vi "41 Config File Write GPS Time (x64-2018).vi"(0 "GPS Time":string, 5 "GPS Date":string, 7 "Labview Time":dbl=0.1, 9 "CPU Time":dbl=0.1, 11 "Tick Count":dbl=0.1, 12 "GPS Lock":bool) -> ()   [LabVIEW 2017]
uses:
  <vilib>/Utility/config.llb/Write Key (Double).vi
  <vilib>/Utility/config.llb/Write Key (String).vi
  <vilib>/Utility/config.llb/Write Key (Boolean).vi
  <vilib>/Utility/config.llb/NI_LVConfig.lvlib
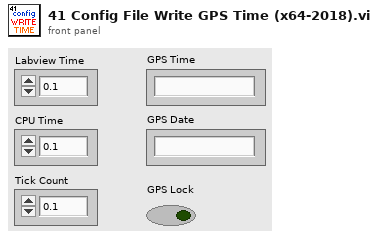
[diagram p1: front panel]
types:
  T1 = typedef "NI_LVConfig.lvlib/Config Data RefNum.ctl" = refnum<k1>
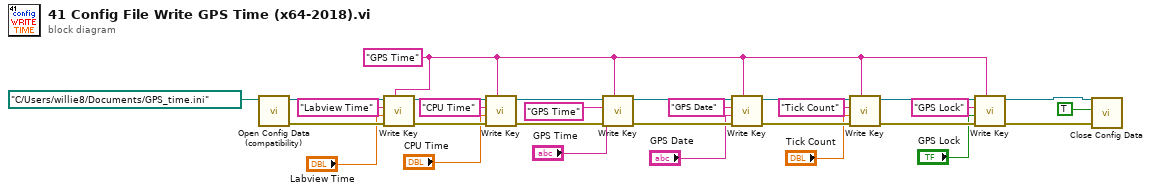
[diagram p0: block diagram]
diagram:
  w3 = "GPS Time" ("section")
  n1 = call <vilib>:"Open Config Data (compatibility).vi"("configuration file path"=path "C:/Users/willie8/Documents/GPS_time.ini") -> ("error out"=w28:errorcluster, "refnum"=w29:T1)  [unwired: 8 in, 1 out]
  n2 = call-poly <vilib>:"Write Key.vi"("section"=w3, "error in (no error)"=w28, "value"="Labview Time", "key"="Labview Time", "refnum"=w29) -> ("error out"=w23:errorcluster, "refnum out"=w26:T1)  [unwired: 4 in, 1 out]
  n3 = call-poly <vilib>:"Write Key.vi"("section"=w3, "error in (no error)"=w23, "value"="CPU Time", "key"="CPU Time", "refnum"=w26) -> ("error out"=w20:errorcluster, "refnum out"=w21:T1)  [unwired: 4 in, 1 out]
  n4 = call-poly <vilib>:"Write Key.vi"("section"=w3, "error in (no error)"=w20, "value"="GPS Time", "key"="GPS Time", "refnum"=w21) -> ("error out"=w17:errorcluster, "refnum out"=w18:T1)  [unwired: 4 in, 1 out]
  n5 = call-poly <vilib>:"Write Key.vi"("section"=w3, "error in (no error)"=w17, "value"="GPS Date", "key"="GPS Date", "refnum"=w18) -> ("error out"=w13:errorcluster, "refnum out"=w14:T1)  [unwired: 4 in, 1 out]
  n6 = call-poly <vilib>:"Write Key.vi"("section"=w3, "error in (no error)"=w13, "value"="Tick Count", "key"="Tick Count", "refnum"=w14) -> ("error out"=w7:errorcluster, "refnum out"=w8:T1)  [unwired: 4 in, 1 out]
  n7 = call-poly <vilib>:"Write Key.vi"("section"=w3, "error in (no error)"=w7, "value"="GPS Lock", "key"="GPS Lock", "refnum"=w8) -> ("error out"=w6:errorcluster, "refnum out"=w5:T1)  [unwired: 4 in, 1 out]
  n8 = call <vilib>:"Close Config Data.vi"("error in (no error)"=w6, "write file if changed (T)"=TRUE ("write configuration file? (T)"), "refnum"=w5) -> ()  [unwired: 7 in, 2 out]
